vi "test Separate Tx and Rx.vi"(8 "error in (no error)":errorcluster, 11 "TestCase in":refnum<class "Configuration Tests.lvclass">) -> (0 "error out":errorcluster, 3 "TestCase out":refnum<class "Configuration Tests.lvclass">)   [LabVIEW 2017, in "Configuration Tests.lvclass"]
uses:
  Configuration Tests.lvclass
  Mock Classes/Transfer Group/Mock Transfer Group.lvclass
  C:/Git/DSF/Data Sharing Framework Core/Classes/Transfer Group/Transfer Group.lvclass
  Typedefs/DSF Direction.ctl
  Classes/Transfer Group/Transfer Group.lvclass/Transfer Group.ctl
  <vilib>/addons/_JKI Toolkits/VI Tester/TestCase.llb/TestCase.lvclass
  Classes/Transfer Group/Transfer Group.lvclass
  DSF Core.lvlib
  C:/Program Files (x86)/National Instruments/LabVIEW 2017/vi.lib/addons/_JKI Toolkits/VI Tester/TestCase.llb/TestCase.lvclass
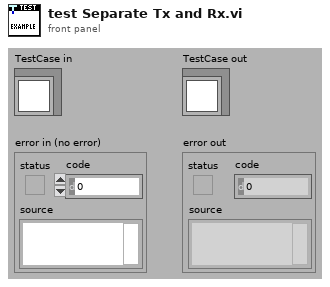
[diagram p1: front panel]
types:
  T1 = typedef "DSF Core.lvlib/DSF Direction.ctl" = enum8{"Tx", "Rx"}
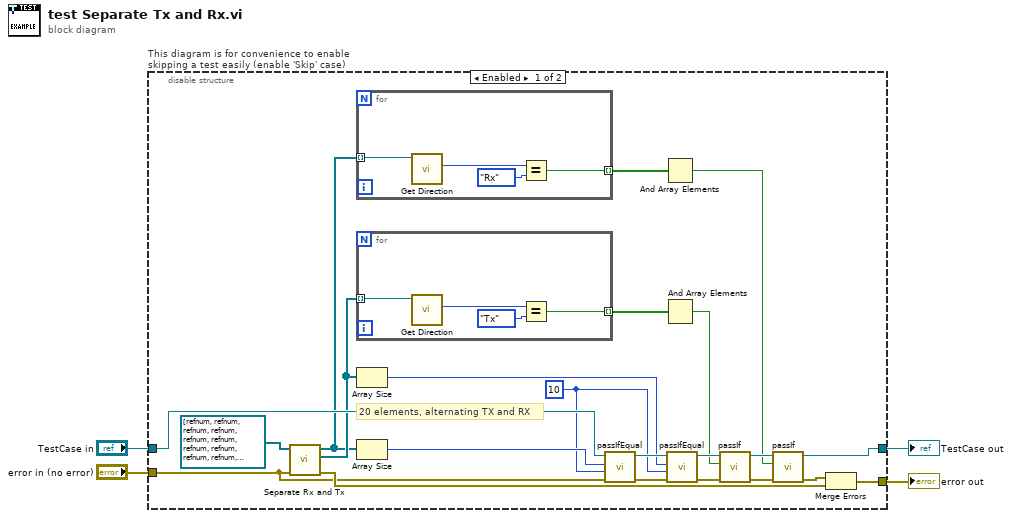
[diagram p0: block diagram]
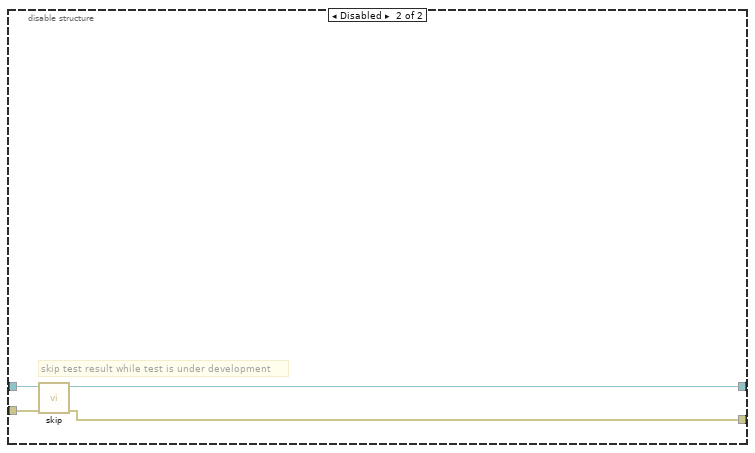
[diagram p2: hidden frame]
diagram:
  n1 = disable-structure "This diagram is for convenience to enable skipping a test easily (enable 'Skip' case)" shown="Enabled" {
    disable-tunnel: "TestCase in" -> [w24 w38]
    disable-tunnel: [w10 w36] -> w1
    disable-tunnel: [w6 w37] -> w3
    disable-tunnel: "error in (no error)" -> [w5 w35]
    frame Enabled {
      w20 = 10 ("size(s)")
      # "20 elements, alternating TX and RX"
      n2 = call "Separate Rx and Tx.vi"("error in (no error)"=w5, "Transfer Groups"=refnum<class "Mock Transfer Group.lvclass">[] [refnum, refnum, refnum, refnum, refnum, refnum, refnum, refnum, refnum, refnum, refnum, refnum, refnum, refnum, refnum, refnum, refnum, refnum, refnum, refnum] ("interleaved array")) -> ("error out"=w7:errorcluster, "Tx Transfer Groups"=w18:refnum<class "Transfer Group.lvclass">[], "Rx Transfer Groups"=w15:refnum<class "Transfer Group.lvclass">[])  [unwired: 7 in]
      n3 = for {
        tunnel: w15 -> [w30] mode=indexing
        tunnel: [w27] -> w16 mode=indexing
        n4 = call "Get Direction.vi"("Transfer Group in"=w30) -> ("Direction"=w29:T1)  [unwired: 9 in, 1 out]
        n5 = Equal?(x=w29, y=DSF_Direction."Rx") -> (x = y?=w27:bool)
      }
      n6 = for {
        tunnel: w18 -> [w34] mode=indexing
        tunnel: [w31] -> w17 mode=indexing
        n7 = call "Get Direction.vi"("Transfer Group in"=w34) -> ("Direction"=w33:T1)  [unwired: 9 in, 1 out]
        n8 = Equal?(x=w33, y=DSF_Direction."Tx") -> (x = y?=w31:bool)
      }
      n9 = Array Size(array=w18) -> (size(s)=w19:i32)
      n10 = Array Size(array=w15) -> (size(s)=w23:i32)
      n11 = call-dynamic "passIfEqual.vi"("error in (no error)"=w5, "y"=w20, "x"=w23, "TestCase in"=w24) -> ("error out"=w25:errorcluster, "TestCase out"=w21:refnum<class "Configuration Tests.lvclass">)  [unwired: 6 in]
      n12 = And Array Elements(Boolean array=w16) -> (logical AND=w9:bool)
      n13 = And Array Elements(Boolean array=w17) -> (logical AND=w12:bool)
      n14 = call-dynamic "passIfEqual.vi"("error in (no error)"=w25, "y"=w20, "x"=w19, "TestCase in"=w21) -> ("error out"=w22:errorcluster, "TestCase out"=w13:refnum<class "Configuration Tests.lvclass">)  [unwired: 6 in]
      n15 = call-dynamic "passIf.vi"("error in (no error)"=w22, "pass"=w12, "TestCase in"=w13) -> ("error out"=w14:errorcluster, "TestCase out"=w11:refnum<class "Configuration Tests.lvclass">)  [unwired: 7 in]
      n16 = call-dynamic "passIf.vi"("error in (no error)"=w14, "pass"=w9, "TestCase in"=w11) -> ("error out"=w8:errorcluster, "TestCase out"=w10:refnum<class "Configuration Tests.lvclass">)  [unwired: 7 in]
      n17 = Merge Errors(w8, w7) -> (w6:errorcluster)
    }
    frame Disabled {
      # "skip test result while test is under development"
      n18 = call <vilib>:"skip.vi"("error in (no error)"=w35, "TestCase in"=w38) -> ("error out"=w37:errorcluster, "TestCase out"=w36:refnum<class "Configuration Tests.lvclass">)  [unwired: 8 in]
    }
  }
  "error out" <- w3
  "TestCase out" <- w1
